vi "ObjDet_Read_Dataset_All.vi"(0 "Train Image Path":path, 5 "Train Anno Path":path, 7 "Test Image Path":path, 9 "Test Anno Path":path, 11 "error in (no error)":errorcluster, 12 "Dims(C,H,W)":T1={"C"=-1, "H"=-1, "W"=-1}) -> (4 "Dataset":T2={"Train"={"Inputs Ref."=variant(refnum<data-value> refnum), "Dataset_Size"=0, "Dims_In"={"C"=0, "H"=0, "W"=0}, "Outputs Refs"=refnum, "No of Classes "=0, "Labels"=["large", "small"], "File Paths"=[]}, "Validation"={"Inputs Ref."=variant(refnum<data-value> refnum), "Dataset_Size"=0, "Dims_In"={"C"=0, "H"=0, "W"=0}, "Outputs Refs"=refnum, "No of Classes "=0, "Labels"=["large", "small"], "File Paths"=[]}, "Test"={"Inputs Ref."=variant(refnum<data-value> refnum), "Dataset_Size"=0, "Dims_In"={"C"=0, "H"=0, "W"=0}, "Outputs Refs"=refnum, "No of Classes "=0, "Labels"=["large", "small"], "File Paths"=[]}}, 6 "Anchors":dbl[][](array[numeric]), 15 "error out":errorcluster)   [LabVIEW 2020]
uses:
  <vilib>/Ngene/Deep Learning Toolkit/Toolkit/NN_Data/API/DataSet/DataSet_Types/NN_DataSets_All(In3D_OutBBox).ctl
  <vilib>/Ngene/Deep Learning Toolkit/Toolkit/NN_Data/API/DataSet/DataSet_Types/NN_DataSet(In3D_OutBBox).ctl
  <vilib>/Ngene/Deep Learning Toolkit/Toolkit/NN_Data/API/NN_Dims(C,H,W).ctl
  <vilib>/Ngene/Deep Learning Toolkit/Toolkit/NN_Data/Controls/DataRef_Types/1D/NN_Data_ref(1D_BBox).ctl
  <vilib>/Ngene/Deep Learning Toolkit/Toolkit/NN_Data/API/Data/Detection_Types/NN_Image_Annotations.ctl
  <vilib>/Ngene/Deep Learning Toolkit/Toolkit/NN_Data/API/Data/Detection_Types/NN_BBox_Annotation.ctl
  <vilib>/Ngene/Deep Learning Toolkit/Toolkit/NN_Data/API/Data/Detection_Types/NN_BBox.ctl
  <vilib>/Ngene/Deep Learning Toolkit/Toolkit/Deep_Learning_Toolkit_by_Ngene.lvlib
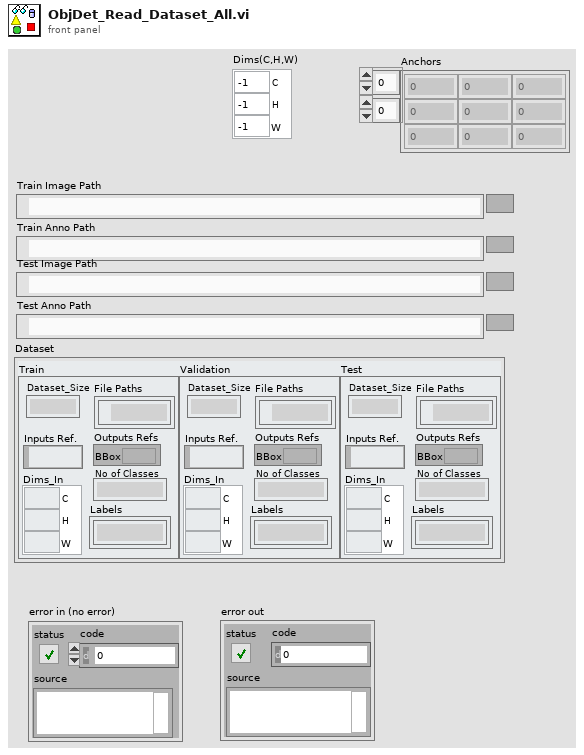
[diagram p1: front panel]
types:
  T1 = typedef "Deep_Learning_Toolkit_by_Ngene.lvlib/NN_Dims(C,H,W).ctl" = cluster{"C":i32, "H":i32, "W":i32}
  T2 = typedef "Deep_Learning_Toolkit_by_Ngene.lvlib/NN_DataSets_All(In3D_OutBBox).ctl" = cluster{"Train":T3, "Validation":T3, "Test":T3}
  T3 = typedef "Deep_Learning_Toolkit_by_Ngene.lvlib/NN_DataSet(In3D_OutBBox).ctl" = cluster{"Inputs Ref.":variant, "Dataset_Size":i32, "Dims_In":T1, "Outputs Refs":T4, "No of Classes ":i32, "Labels":string[], "File Paths":path[]}
  T4 = typedef "Deep_Learning_Toolkit_by_Ngene.lvlib/NN_Data_ref(1D_BBox).ctl" = refnum<data-value>
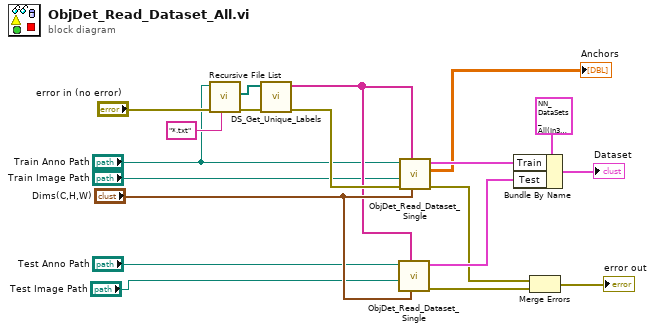
[diagram p0: block diagram]
diagram:
  n1 = call <vilib>:"Recursive File List.vi"("pattern"="*.txt", "error in (no error)"="error in (no error)", "Folder Path"="Train Anno Path") -> ("error out"=w16:errorcluster, "All Files in Dir"=w13:path[])  [unwired: 4 in, 3 out]
  n2 = call "DS_Get_Unique_Labels.vi"("error in (no error)"=w16, "Anno File Paths"=w13) -> ("error out"=w15:errorcluster, "Unique labels"=w10:string[])  [unwired: 8 in]
  n3 = call "ObjDet_Read_Dataset_Single.vi"("Dims(C,H,W)"="Dims(C,H,W)", "Unique labels"=w10, "Dataset Path (Images)"="Test Image Path", "Annotations Path"="Test Anno Path") -> ("error out"=w4:errorcluster, "NN_DataSet(In3D_OutBBox)"=w11:T3)  [unwired: 5 in, 1 out]
  n4 = call "ObjDet_Read_Dataset_Single.vi"("Dims(C,H,W)"="Dims(C,H,W)", "Unique labels"=w10, "error in (no error)"=w15, "Dataset Path (Images)"="Train Image Path", "Annotations Path"="Train Anno Path") -> ("error out"=w5:errorcluster, "Anchors"=→"Anchors":dbl[][], "NN_DataSet(In3D_OutBBox)"=w14:T3)  [unwired: 4 in]
  n5 = Bundle By Name(cluster=T2 {"Train"={"Inputs Ref."=variant(refnum<data-value> refnum), "Dataset_Size"=0, "Dims_In"={"C"=0, "H"=0, "W"=0}, "Outputs Refs"=refnum, "No of Classes "=0, "Labels"=["large", "small"], "File Paths"=[]}, "Validation"={"Inputs Ref."=variant(refnum<data-value> refnum), "Dataset_Size"=0, "Dims_In"={"C"=0, "H"=0, "W"=0}, "Outputs Refs"=refnum, "No of Classes "=0, "Labels"=["large", "small"], "File Paths"=[]}, "Test"={"Inputs Ref."=variant(refnum<data-value> refnum), "Dataset_Size"=0, "Dims_In"={"C"=0, "H"=0, "W"=0}, "Outputs Refs"=refnum, "No of Classes "=0, "Labels"=["large", "small"], "File Paths"=[]}} ("Dataset_Refs_All(In3D_OutBBox)"), "Train"=w14, "Test"=w11) -> (→"Dataset":T2)
  n6 = Merge Errors(w5, w4) -> (→"error out":errorcluster)
